vi "Move Right.vi"(5 "Label":string="Test", 6 "Make Vertical":bool=TRUE, 7 "Goal":T3, 8 "error in":errorcluster, 9 "Speed":dbl=25.0, 10 "Mask":string="Relative", 11 "Location":string="Base") -> (0 "error out":errorcluster, 1 "Speed Out":dbl=-25.0, 2 "Mask Out":string="Relative", 3 "Location Out":string=" ", 4 "Current":T2)   [LabVIEW 2013]
uses:
  <vilib>/Analysis/Matrix/Datatypes/RealMatrix.ctl
  Arm Globals.vi
  <vilib>/Analysis/Matrix/Numeric/Multiply/Multiply - RM,RM.vi
  ROS/Code/Console/Servers/ServerSubs/(nist) Arm Globals.vi
  <vilib>/Analysis/Matrix/NI_Matrix.lvlib
panel:
  out "XYZOAT":T1
  out "Joints":dbl[][](array[numeric]) format="%.1f"
  out "Start":T2 format="%.1f"
  out "T":T2 format="%.3f"
  out "Int Pose":T2 format="%.1f"
  out "End Pose":T2 format="%.1f"
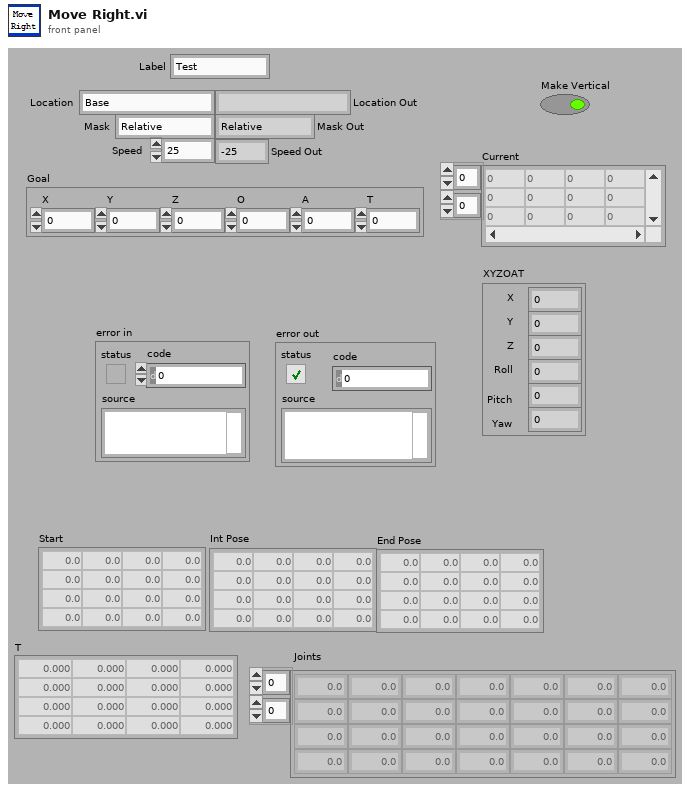
[diagram p1: front panel]
types:
  T1 = cluster{"X":dbl, "Y":dbl, "Z":dbl, "Roll":dbl, "Pitch":dbl, "Yaw":dbl}
  T2 = typedef "NI_Matrix.lvlib/RealMatrix.ctl" = dbl[][]
  T3 = cluster{"X":dbl, "Y":dbl, "Z":dbl, "O":dbl, "A":dbl, "T":dbl}
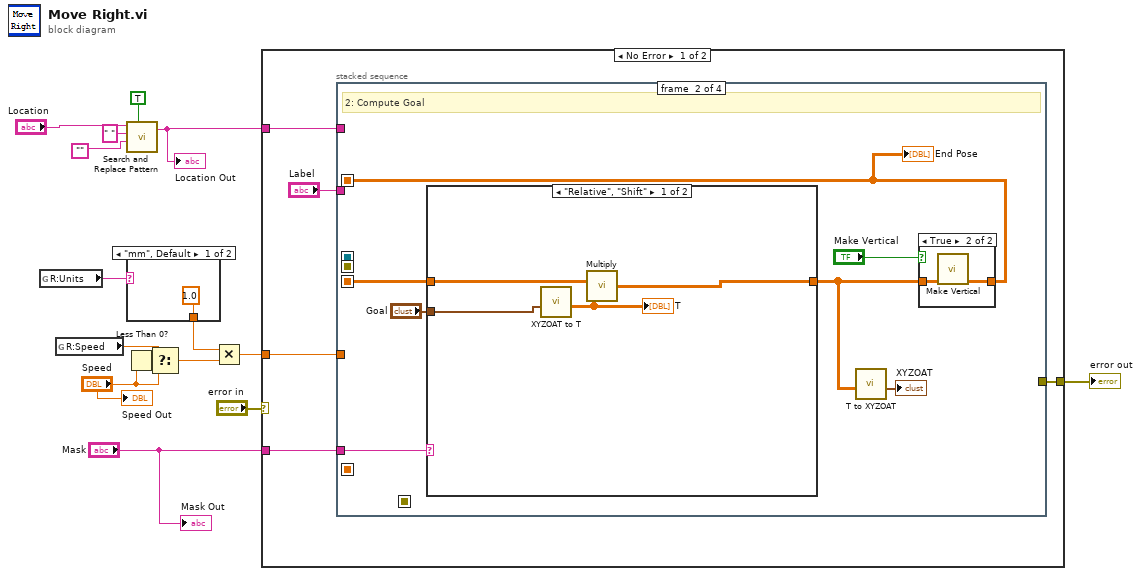
[diagram p0: block diagram]
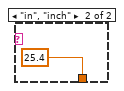
[diagram p2: hidden frame]
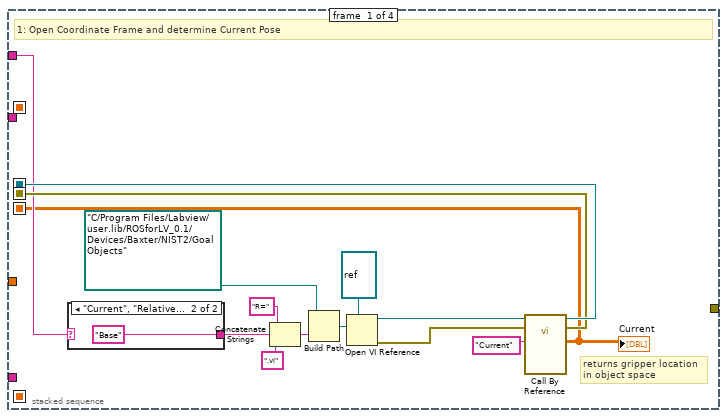
[diagram p3: hidden frame]
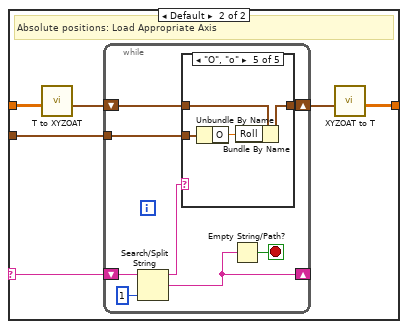
[diagram p5: hidden frame]
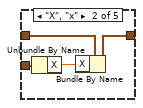
[diagram p7: hidden frame]
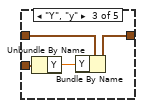
[diagram p8: hidden frame]
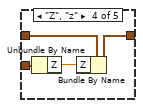
[diagram p9: hidden frame]
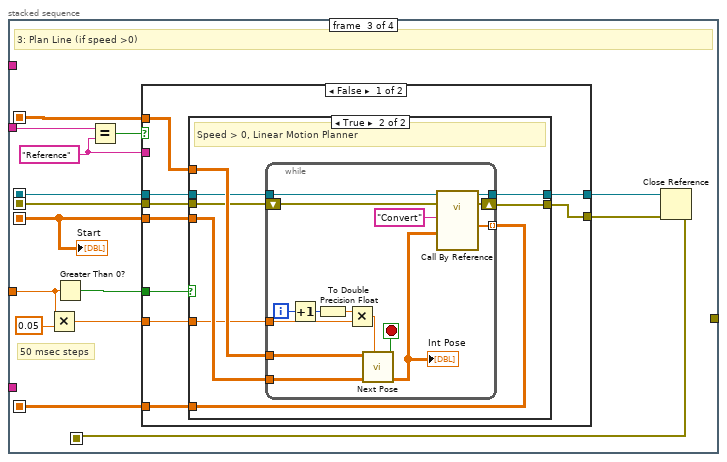
[diagram p11: hidden frame]
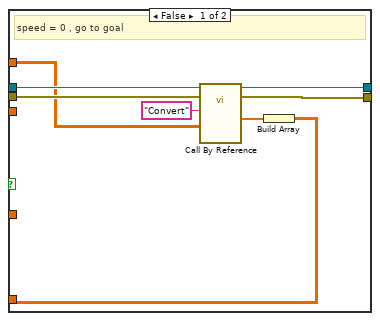
[diagram p12: hidden frame]
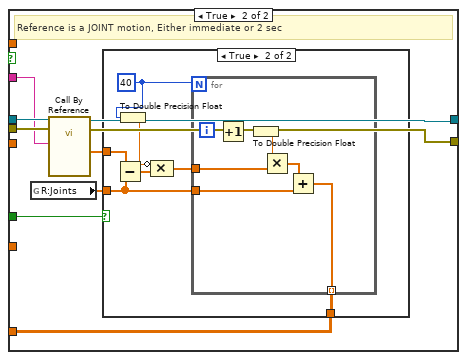
[diagram p13: hidden frame]
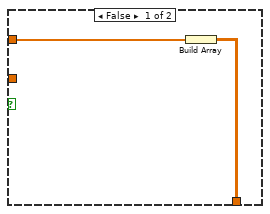
[diagram p14: hidden frame]
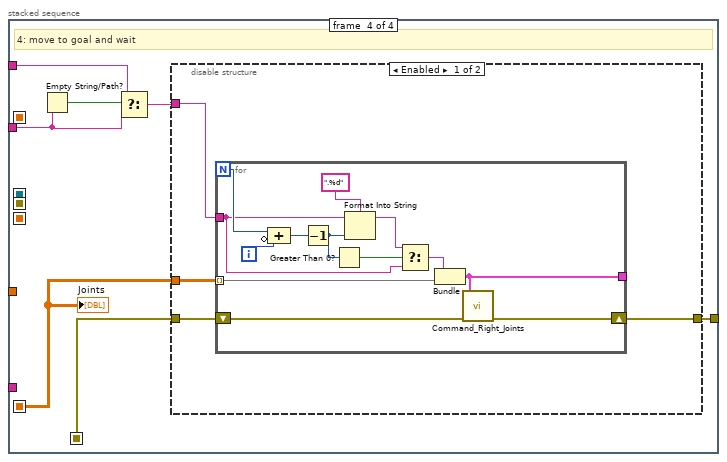
[diagram p15: hidden frame]
diagram:
  n1 = global read "Arm Globals.vi" "R:Units"() -> (w11:string)
  n2 = global read "Arm Globals.vi" "R:Speed"() -> (w12:dbl)
  n3 = Less Than 0?(x="Speed") -> (x < 0?=w13:bool)
  n4 = call <vilib>:"Search and Replace Pattern.vi"("string"="Location", "regular expression (\"\")"=" " ("regular expression (\"\")"), "replace string (\"\")"="", "replace all? (F)"=TRUE) -> ("result string"=w1:string)  [unwired: 1 in, 1 out]
  "Location Out" <- w1
  n5 = case shown="\"mm\", Default" w11 {
    tunnel: [1.0 ("x") 25.4 ("x")] -> w8
    frame "mm", Default {
    }
    frame "in", "inch" {
    }
  }
  n6 = Select(t=w12, s=w13, f="Speed") -> (s? t:f=w9:dbl)
  n7 = Multiply(x=w8, y=w9) -> (x*y=w10:dbl)
  n8 = case shown="No Error" "error in" {
    selector: "error in" -> [_ w189]
    tunnel: [w22 w189] -> w14
    tunnel: w1 -> [w20 _]
    tunnel: w10 -> [w19 _]
    tunnel: "Mask" -> [w18 _]
    frame No Error {
      n9 = stacked-sequence {
        seq-local: [w26 _ _ _] -> [_ _ w94 _]
        seq-local: [w25 _ _ _] -> [_ _ w93 _]
        seq-local: [w23 _ _ _] -> [_ w44 w86 _]
        seq-local: [_ w41 _ _] -> [_ _ w87 _]
        seq-local: [_ _ w95 _] -> [_ _ _ w170]
        seq-local: [_ _ w90 _] -> [_ _ _ w169]
        tunnel: [_ _ _ w168] -> w22
        tunnel: w20 -> [w24 _ _ w165]
        tunnel: "Label" -> [_ _ w88 w164]
        tunnel: w19 -> [_ _ w84 _]
        tunnel: w18 -> [_ w42 _ _]
        frame #0 {
          # "returns gripper location\nin object space"
          # "1: Open Coordinate Frame and determine Current Pose"
          n10 = case shown="\"Current\", \"Relative\"" w24 {
            selector: w24 -> [w37 _]
            tunnel: [w37 "Base"] -> w30
            frame Default {
            }
            frame "Current", "Relative" {
            }
          }
          n11 = Concatenate Strings("R=", w30, ".vi" ("string")) -> (w34:string)
          n12 = Build Path(base path=path "C:/Program Files/Labview/user.lib/ROSforLV_0.1/Devices/Baxter/NIST2/Goal Objects", name or relative path=w34) -> (appended path=w35:path)
          n13 = Open VI Reference(type specifier VI Refnum (for type only)=refnum<vi> refnum, vi path=w35) -> (vi reference=w28:refnum<vi>, error out=w27:errorcluster)  [unwired: 4 in]
          n14 = call-by-ref "?"(reference=w28, error in=w27, "Command"="Current") -> (reference out=w26:refnum<vi>, error out=w25:errorcluster, "Matrix"=w23:T2)  [unwired: 8 in, 2 out]
          "Current" <- w23
        }
        frame #1 {
          # "2: Compute Goal"
          n15 = case shown="\"Relative\", \"Shift\"" w42 {
            selector: w42 -> [_ w55]
            tunnel: [w47 w50] -> w39
            tunnel: w44 -> [w49 w53]
            tunnel: "Goal" -> [w46 w54]
            frame "Relative", "Shift" {
              n16 = call "XYZOAT to T.vi"("XYZOAT"=w46) -> ("T"=w48:T2)  [unwired: 10 in]
              "T" <- w48
              n17 = call-poly <vilib>:"Multiply.vi"("Real Matrix B"=w48, "Real Matrix A"=w49) -> ("A * B"=w47:T2)
            }
            frame Default {
              # "Absolute positions: Load Appropriate Axis"
              n18 = call "T to XYZOAT.vi"("T"=w53) -> ("XYZOAT"=w52:T1)  [unwired: 10 in]
              n19 = while {
                shift-right: [w56] -> _
                shift-left: w55 -> [w63]
                shift-right: [w57] -> w51
                shift-left: w52 -> [w58]
                tunnel: w54 -> [w59]
                stop <- w61 stop-if-true
                n20 = Search/Split String(string=w63, offset (0)=1) -> (substring before match=w60:string, match + rest of string=w56:string)  [unwired: 1 in, 1 out]
                n21 = case shown="\"O\", \"o\"" w60 {
                  tunnel: w59 -> [_ w68 w72 w76 w80]
                  tunnel: w58 -> [w64 w66 w70 w74 w78]
                  tunnel: [w64 w65 w69 w73 w77] -> w57
                  frame Default {
                  }
                  frame "X", "x" {
                    n22 = Unbundle By Name(w68) -> ("X"=w67:dbl)
                    n23 = Bundle By Name(cluster=w66, "X"=w67) -> (w65:T1)
                  }
                  frame "Y", "y" {
                    n24 = Unbundle By Name(w72) -> ("Y"=w71:dbl)
                    n25 = Bundle By Name(cluster=w70, "Y"=w71) -> (w69:T1)
                  }
                  frame "Z", "z" {
                    n26 = Unbundle By Name(w76) -> ("Z"=w75:dbl)
                    n27 = Bundle By Name(cluster=w74, "Z"=w75) -> (w73:T1)
                  }
                  frame "O", "o" {
                    n28 = Unbundle By Name(w80) -> ("O"=w79:dbl)
                    n29 = Bundle By Name(cluster=w78, "Roll"=w79) -> (w77:T1)
                  }
                }
                n30 = Empty String/Path?(string/path=w56) -> (empty?=w61:bool)
              }
              n31 = call "XYZOAT to T.vi"("XYZOAT"=w51) -> ("T"=w50:T2)  [unwired: 10 in]
            }
          }
          n32 = call "T to XYZOAT.vi"("T"=w39) -> ("XYZOAT"=→"XYZOAT":T1)  [unwired: 10 in]
          n33 = case shown="True" "Make Vertical" {
            tunnel: w39 -> [w81 w83]
            tunnel: [w81 w82] -> w41
            frame False {
            }
            frame True {
              n34 = call "Make Vertical.vi"("Matrix"=w83) -> ("Vertical Matrix"=w82:T2)  [unwired: 10 in]
            }
          }
          "End Pose" <- w41
        }
        frame #2 {
          w85 = "Reference" ("y")
          # "50 msec steps"
          # "3: Plan Line (if speed >0)"
          n35 = Multiply(x=w84, y=0.05) -> (x*y=w96:dbl)
          n36 = Greater Than 0?(x=w84) -> (x > 0?=w97:bool)
          n37 = Equal?(x=w88, y=w85) -> (x = y?=w89:bool)
          n38 = case shown="False" w89 {
            tunnel: w97 -> [w107 w140]
            tunnel: w86 -> [w106 _]
            tunnel: w87 -> [w105 _]
            tunnel: w96 -> [w104 _]
            tunnel: [w103 w142] -> w95
            tunnel: w94 -> [w102 w147]
            tunnel: w93 -> [w101 w146]
            tunnel: [w100 w145] -> w92
            tunnel: [w99 w144] -> w91
            tunnel: w85 -> [_ w141]
            frame False {
              n39 = case shown="True" w107 {
                tunnel: w106 -> [_ w123]
                tunnel: w105 -> [w112 w122]
                tunnel: w104 -> [_ w121]
                tunnel: [w108 w116] -> w103
                tunnel: w102 -> [w114 w120]
                tunnel: w101 -> [w113 w119]
                tunnel: [w111 w118] -> w100
                tunnel: [w110 w117] -> w99
                frame False {
                  # "speed = 0 , go to goal"
                  n40 = call-by-ref "?"(reference=w114, error in=w113, "Matrix"=w112, "Command"="Convert") -> (reference out=w111:refnum<vi>, error out=w110:errorcluster, "Joints"=w109:dbl[])  [unwired: 7 in, 2 out]
                  n41 = Build Array(w109) -> (w108:dbl[][])
                }
                frame True {
                  # "Speed > 0, Linear Motion Planner"
                  n42 = while {
                    tunnel: w122 -> [w132]
                    tunnel: w123 -> [w131]
                    tunnel: w121 -> [w134]
                    tunnel: w120 -> [w129]
                    shift-right: [w128] -> w117
                    shift-left: w119 -> [w124]
                    tunnel: [w126] -> w116 mode=indexing
                    tunnel: [w125] -> w118
                    i -> [w137]
                    stop <- w138 stop-if-true
                    n43 = Increment(x=w137) -> (x+1=w135:i32)
                    n44 = To Double Precision Float(number=w135) -> (double precision float=w133:dbl)
                    n45 = Multiply(x=w133, y=w134) -> (x*y=w136:dbl)
                    n46 = call "Next Pose.vi"("Step"=w136, "Start"=w131, "Goal"=w132) -> ("Pose"=w127:T2, "At Goal"=w138:bool)  [unwired: 7 in]
                    "Int Pose" <- w127
                    n47 = call-by-ref "Call By Reference"(reference=w129, error in=w124, "Matrix"=w127, "Command"="Convert") -> (reference out=w125:refnum<vi>, error out=w128:errorcluster, "Joints"=w126:dbl[])  [unwired: 7 in, 2 out]
                  }
                }
              }
            }
            frame True {
              # "Reference is a JOINT motion, Either immediate or 2 sec"
              n48 = global read "(nist) Arm Globals.vi" "R:Joints"() -> (w139:dbl[])
              n49 = call-by-ref "Call By Reference"(reference=w147, error in=w146, "Command"=w141) -> (reference out=w145:refnum<vi>, error out=w144:errorcluster, "Joints"=w143:dbl[])  [unwired: 8 in, 2 out]
              n50 = case shown="True" w140 {
                tunnel: w143 -> [w149 w156]
                tunnel: [w148 w150] -> w142
                tunnel: w139 -> [_ w151]
                frame False {
                  n51 = Build Array(w149) -> (w148:dbl[][])
                }
                frame True {
                  w154 = 40
                  n52 = Subtract(x=w156, y=w151) -> (x-y=w155:dbl[])
                  n53 = To Double Precision Float(number=w154) -> (double precision float=w153:dbl)
                  n54 = Compound Arithmetic op=MULTIPLY(invert w153, w155) -> (w152:dbl[])
                  n55 = for {
                    N: w154 -> [_]
                    tunnel: w152 -> [w161]
                    tunnel: w151 -> [w159]
                    tunnel: [w157] -> w150 mode=indexing
                    i -> [w163]
                    n56 = Increment(x=w163) -> (x+1=w162:i32)
                    n57 = To Double Precision Float(number=w162) -> (double precision float=w160:dbl)
                    n58 = Multiply(x=w160, y=w161) -> (x*y=w158:dbl[])
                    n59 = Add(x=w158, y=w159) -> (x+y=w157:dbl[])
                  }
                }
              }
            }
          }
          n60 = Close Reference(reference=w92, error in (no error)=w91) -> (error out=w90:errorcluster)
          "Start" <- w86
        }
        frame #3 {
          # "4: move to goal and wait"
          n61 = Empty String/Path?(string/path=w164) -> (empty?=w167:bool)
          n62 = Select(t=w165, s=w167, f=w164) -> (s? t:f=w166:string)
          n63 = disable-structure shown="Enabled" {
            disable-tunnel: w170 -> [w174 _]
            disable-tunnel: w169 -> [w173 w188]
            disable-tunnel: [w171 w188] -> w168
            disable-tunnel: w166 -> [w172 _]
            frame Enabled {
              n64 = for {
                N -> [w187]
                tunnel: w172 -> [w178]
                tunnel: w174 -> [w177] mode=indexing
                shift-right: [w183] -> w171
                shift-left: w173 -> [w184]
                tunnel: [w176] -> _
                i -> [w186]
                n65 = Compound Arithmetic op=ADD(w187, invert w186) -> (w182:i32)
                n66 = Decrement(x=w182) -> (x-1=w175:i32)
                n67 = Greater Than 0?(x=w175) -> (x > 0?=w181:bool)
                n68 = Format Into String(format string=".%d", initial string=w178, w175) -> (resulting string=w180:string)  [unwired: 1 in, 1 out]
                n69 = Select(t=w180, s=w181, f=w178) -> (s? t:f=w179:string)
                n70 = Bundle("Label"=w179, "Joints"=w177) -> (w176:cluster{"Label":string, "Joints":dbl[]})  [unwired: 1 in]
                n71 = call "Command_Right_Joints.vi"("error in"=w184, "Goal"=w176) -> ("error out"=w183:errorcluster)  [unwired: 6 in, 1 out]
              }
            }
            frame Disabled {
            }
          }
          "Joints" <- w170
        }
      }
    }
    frame Error {
    }
  }
  "error out" <- w14
  "Mask Out" <- "Mask"
  "Speed Out" <- "Speed"
